vi "SV TDMS Write Octave (N Ch).vi"(0 "tdms file":refnum<k34>, 5 "group name in":string="Octave", 7 "channel names in":string[](array[string]), 9 "octave spectra":T1(array[cluster]), 11 "error in":errorcluster, 13 "octave info":T2[](array[typedef]) {"engineering units" items=["custom..."=0, "V"=1, "A"=21, "C"=30, "pC"=31, "s"=32, "-"=29, "Pa"=2, "N"=20, "g"=3, "m/s^2"=4, "m/s"=5, "m"=6, "mm/s"=12, "mm"=13, "micron/s"=14, "micron"=15, "in/s^2"=7, "in/s"=8, "in"=9, "mil/s"=10, "mil"=11, "rad/s^2"=16, "rad/s"=17, "rad"=18, "deg/s^2"=26, "deg/s"=27, "deg"=28, "RPM"=22, "cycle/s^2"=23, "Hz"=24, "cycle"=25, "strain"=19]; "dB reference" format="%.2e"; "weighting filter" items=["Linear", "A-weighting", "B-weighting", "C-weighting", "ITU-R 468-4", "Dolby", "CCITT", "C-message", "Wb", "Wc", "Wd", "We", "Wf", "Wh", "Wj", "Wk", "Wm", "AES17 20 kHz lowpass", "AES17 40 kHz lowpass", "AES17 20 kHz highpass", "AES17 40 kHz highpass"]}) -> (4 "tdms file out":refnum<k34>, 6 "group name out":string="Octave", 8 "channel names out":string[](array[string]), 15 "error out":errorcluster)   [LabVIEW 2017]
doc: "Writes data to the specified .tdms file in a format specific to the polymorphic instance. Wire data to the <B>scaled signal [EU]</B> input to determine the polymorphic instance to use or manually select the instance."
uses:
  <vilib>/addons/_NISVFA/_Shared subVIs/Controls/svc_Octave Info.ctl
  <vilib>/addons/_NISVFA/_Shared subVIs/Controls/svc_Octave Standard.ctl
  <vilib>/addons/_NISVFA/_Shared subVIs/Controls/svc_Weighting Filter Text Ring.ctl
  <vilib>/addons/_NISVFA/_Shared subVIs/Controls/svc_Engineering Units Text Ring.ctl
  <vilib>/addons/_NISVFA/_Shared subVIs/Controls/LV Datatypes.ctl
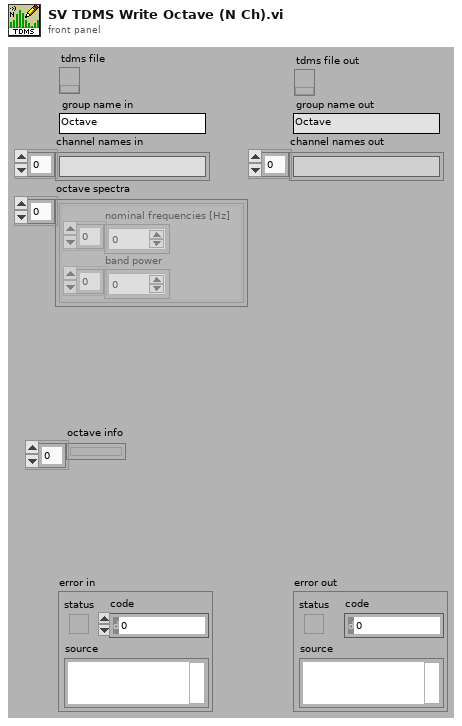
[diagram p1: front panel]
types:
  T1 = cluster{"nominal frequencies [Hz]":dbl[], "band power":dbl[]}[]
  T2 = typedef "svc_Octave Info.ctl" = cluster{"standard":T3, "bandwidth":enum16{"1 octave", "1/3 octave", "1/6 octave", "1/12 octave", "1/24 octave"}, "low band":i32, "high band":i32, "weighting filter":T4, "dB reference":dbl, "dB On":bool, "unit label":string, "channel name":string, "description":string, "engineering units":T5, "custom label":string, "spectrum type":enum16{"power", "magnitude"}, "spectral density":bool, "filters settled":bool}
  T3 = typedef "svc_Octave Standard.ctl" = enum16{"ANSI S1.11", "IEC 61260"}
  T4 = typedef "svc_Weighting Filter Text Ring.ctl" = u16
  T5 = typedef "svc_Engineering Units Text Ring.ctl" = u16
  T6 = typedef "LV Datatypes.ctl" = i32
  T7 = cluster{"nominal frequencies [Hz]":dbl[], "band power":dbl[]}
  T8 = typedef "NI Function Type.ctl" = u16
  T9 = typedef "NI Function SubType.ctl" = u16
  T10 = typedef "svc_X-Axis Units.ctl" = u16
  T11 = cluster{"function type":T8, "function subtype":T9, "X-domain":T10}
  T12 = cluster{"X-axis label":string, "X-unit string":string, "Y-axis label":string, "Y-unit string":string}
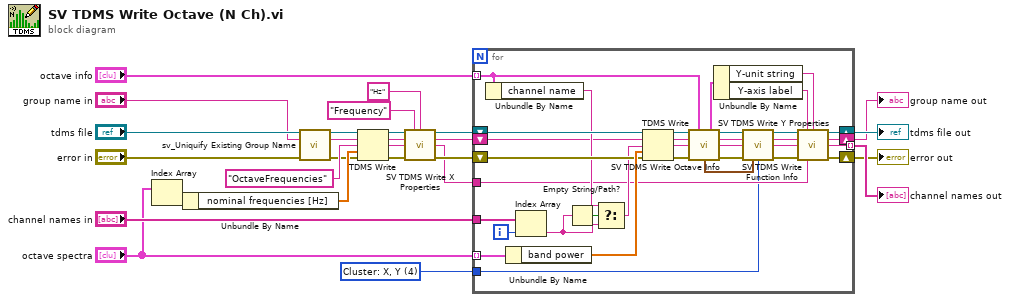
[diagram p0: block diagram]
diagram:
  w1 = T6 4 items=["String: abc"=-2, "Boolean: True or False"=-1, "Scalar: y"=0, "Array: Y"=1, "Waveform: t0, dt, Y, variant"=2, "Cluster: x0, dx, Y"=3, "Cluster: X, Y"=4, "Waterfall"=5, "Colormap"=6] ("LabVIEW datatype")
  n1 = Index Array(array="octave spectra") -> (element=w20:T7)  [unwired: 1 in]
  n2 = Unbundle By Name(w20) -> ("nominal frequencies [Hz]"=w19:dbl[])
  n3 = call <vilib>:"sv_Uniquify Existing Group Name.vi"("tdms file ref"="tdms file", "group name"="group name in", "error in"="error in") -> ("tdms file out"=w16:refnum<k34>, "unique group"=w12:string, "error out"=w13:errorcluster)  [unwired: 10 in]
  n4 = TDMS Write(0:w16, 5:w12, 7:"OctaveFrequencies" ("group name"), 9:w19, 11:w13) -> (4:w11:refnum<k34>, 6:w8:string, 8:w9:string, 15:w10:errorcluster)  [unwired: 1 in]
  n5 = call <vilib>:"SV TDMS Write X Properties.vi"("tdms file in"=w11, "X-axis label"="Frequency" ("channel name"), "X-unit string"="Hz" ("channel name"), "group name"=w8, "channel name"=w9, "error in"=w10) -> ("tdms file out"=w5:refnum<k34>, "group name"=w4:string, "channel name"=w2:string, "error out"=w3:errorcluster)  [unwired: 6 in]
  n6 = for {
    tunnel: "channel names in" -> [w56]
    tunnel: "octave info" -> [w48] mode=indexing
    tunnel: "octave spectra" -> [w60] mode=indexing
    tunnel: [w34] -> w23 mode=indexing
    shift-right: [w33] -> w18
    shift-left: w3 -> [w59]
    shift-right: [w36] -> w27
    shift-left: w5 -> [w58]
    shift-right: [w35] -> w24
    shift-left: w4 -> [w53]
    tunnel: w2 -> [w45]
    tunnel: w1 -> [w28]
    i -> [w51]
    n7 = Unbundle By Name(w48) -> ("channel name"=w55:string)
    n8 = Unbundle By Name(w60) -> ("band power"=w61:dbl[])
    n9 = Index Array(array=w56, index=w51) -> (element=w52:string)
    n10 = Empty String/Path?(string/path=w52) -> (empty?=w57:bool)
    n11 = Select(t=w55, s=w57, f=w52) -> (s? t:f=w54:string)
    n12 = TDMS Write(0:w58, 5:w53, 7:w54, 9:w61, 11:w59) -> (4:w50:refnum<k34>, 6:w47:string, 8:w46:string, 15:w49:errorcluster)  [unwired: 1 in]
    n13 = call <vilib>:"SV TDMS Write Octave Info.vi"("tdms file"=w50, "octave info"=w48, "group name in"=w47, "channel name in"=w46, "error in"=w49) -> ("tdms file out"=w44:refnum<k34>, "group name out"=w43:string, "channel name out"=w42:string, "function info"=w32:T11, "unit info"=w31:T12, "error out"=w41:errorcluster)  [unwired: 5 in]
    n14 = Unbundle By Name(w31) -> ("Y-unit string"=w29:string, "Y-axis label"=w30:string)
    n15 = call <vilib>:"SV TDMS Write Function Info.vi"("tdms file in"=w44, "function info"=w32, "LabVIEW datatype"=w28, "group name"=w43, "channel name"=w42, "error in (no error)"=w41) -> ("tdms file out"=w37:refnum<k34>, "group name out"=w38:string, "channel name out"=w39:string, "error out"=w40:errorcluster)  [unwired: 6 in]
    n16 = call <vilib>:"SV TDMS Write Y Properties.vi"("tdms file"=w37, "y-axis label"=w30, "y-unit string"=w29, "group name"=w38, "channel name"=w39, "error in (no error)"=w40, "xchannel name"=w45) -> ("tdms file out"=w36:refnum<k34>, "group name"=w35:string, "channel name"=w34:string, "error out"=w33:errorcluster)  [unwired: 5 in]
  }
  "error out" <- w18
  "tdms file out" <- w27
  "group name out" <- w24
  "channel names out" <- w23
